vi "LifeTesting.vi"() -> ()   [LabVIEW 2016]
uses:
  <vilib>/Instr/_visa.llb/VISA Configure Serial Port (Instr).vi
  <vilib>/Utility/config.llb/Read Key (Double).vi
  <vilib>/Utility/file.llb/Write Delimited Spreadsheet (DBL).vi
  <vilib>/Utility/config.llb/NI_LVConfig.lvlib
panel:
  in  "两次测量间工作次数":i32=44
  in  "osc chn":i32[](array[numeric])
  in  "总共需要测量次数":i32
  out "轴向声压分布":cluster{dbl[], dbl[]}(graph)
  in  "sensitivity":dbl=0.2
  out "preasure":dbl
  in  "record cycles":dbl=7.0
  in  "freq (MHz)":dbl=1.367
  in  "cycles":dbl=60.0
  in  "Port":u32=12321
  in  "HIFU IP":string="192.168.1.24"
  in  "探头测量中心位置":dbl[][](array[numeric])
  in  "KYCT":refnum<visa-resource-name>
  in  "osc in":refnum<visa-resource-name>
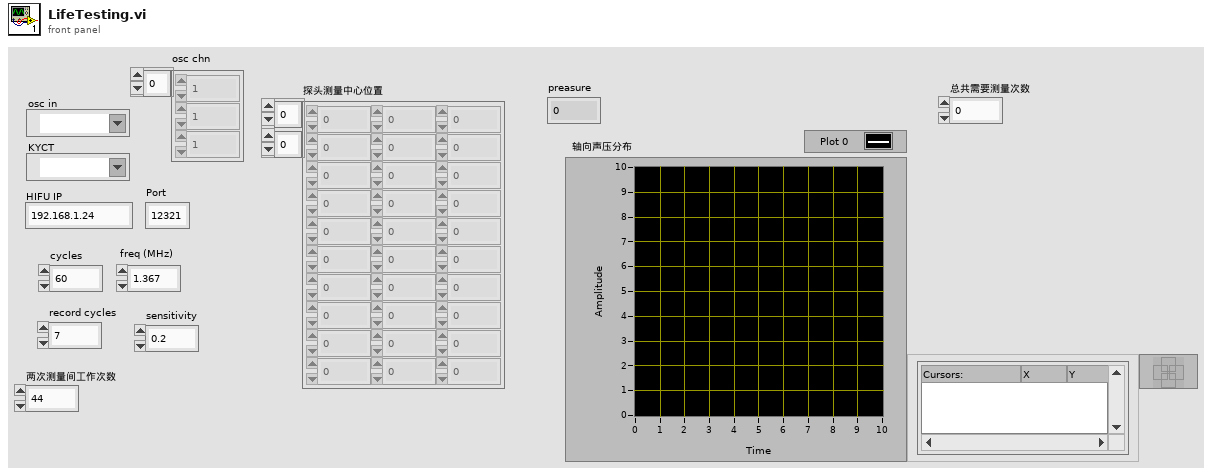
[diagram p1: front panel]
types:
  T1 = typedef "NI_LVConfig.lvlib/Config Data RefNum.ctl" = refnum<k1>
  T2 = typedef "NI_Matrix.lvlib/RealMatrix.ctl" = dbl[][]
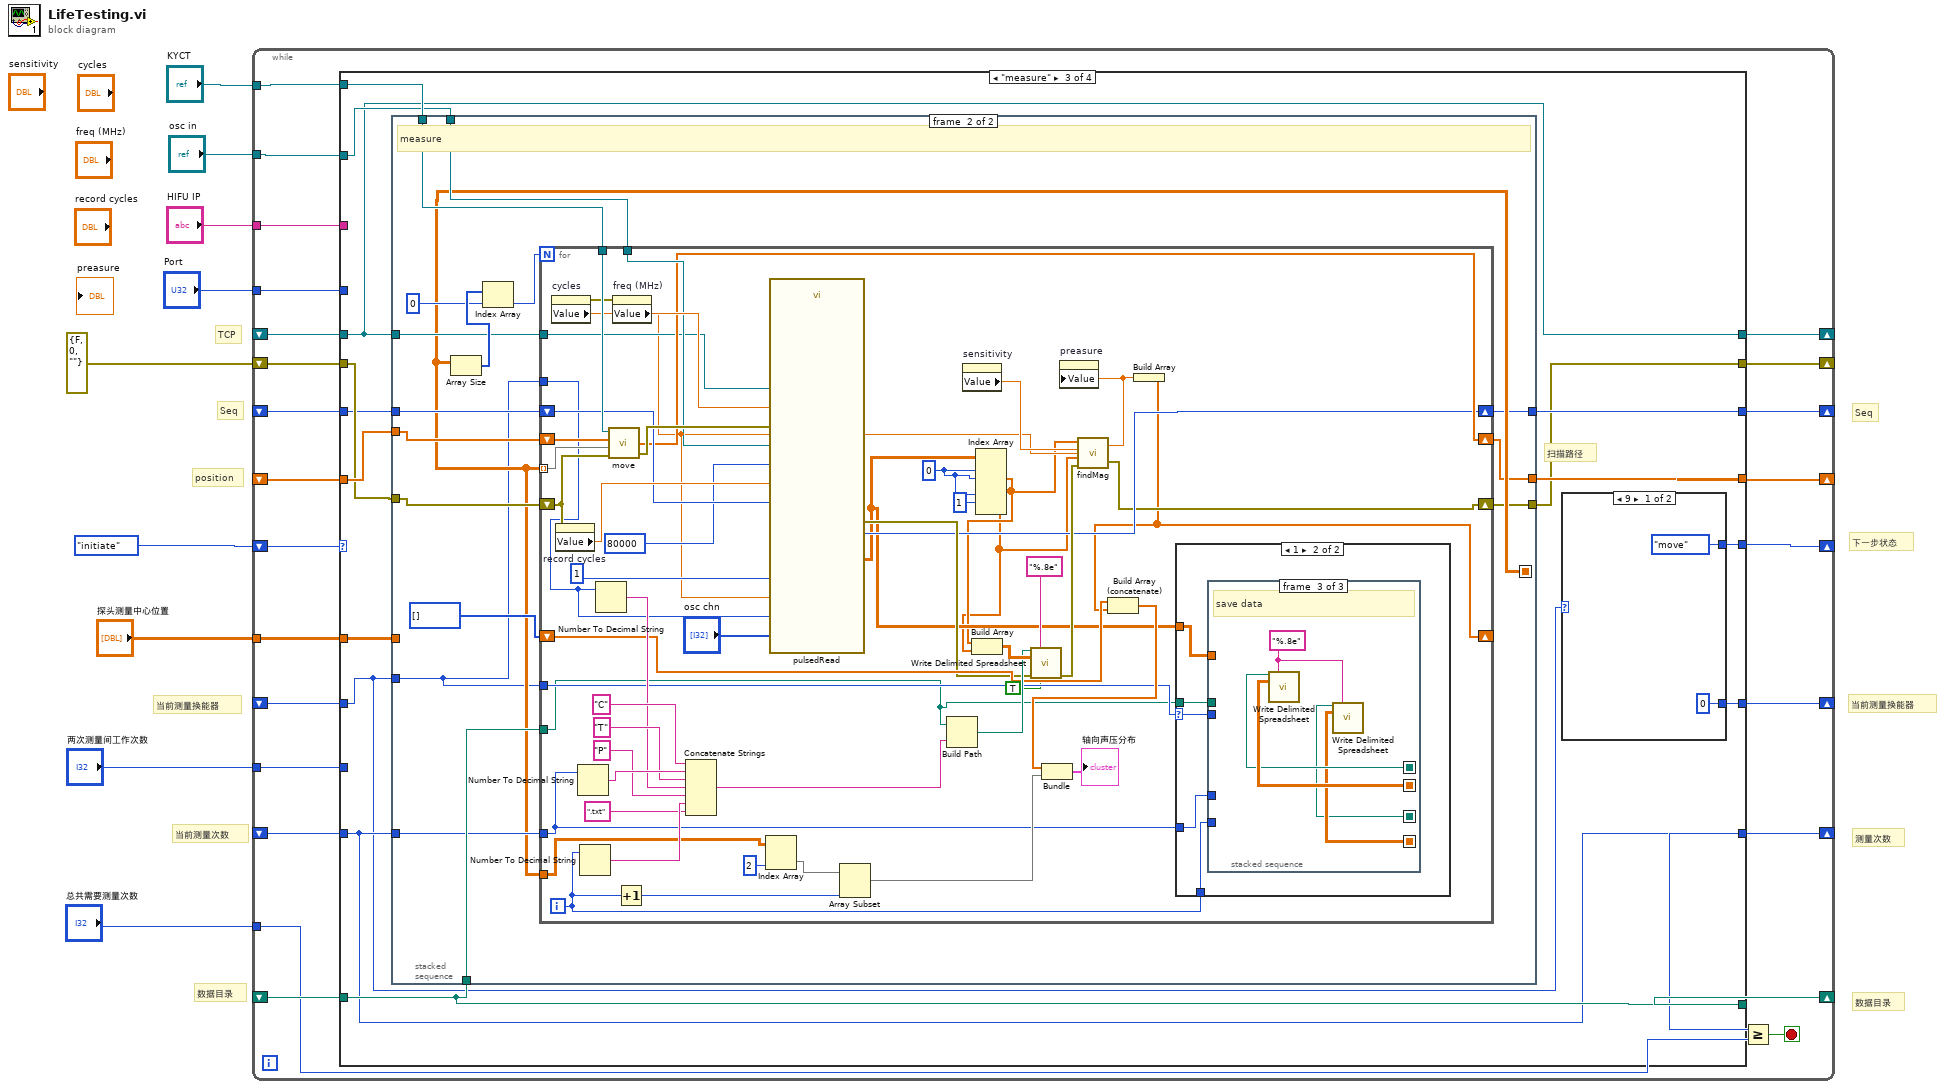
[diagram p0: block diagram]
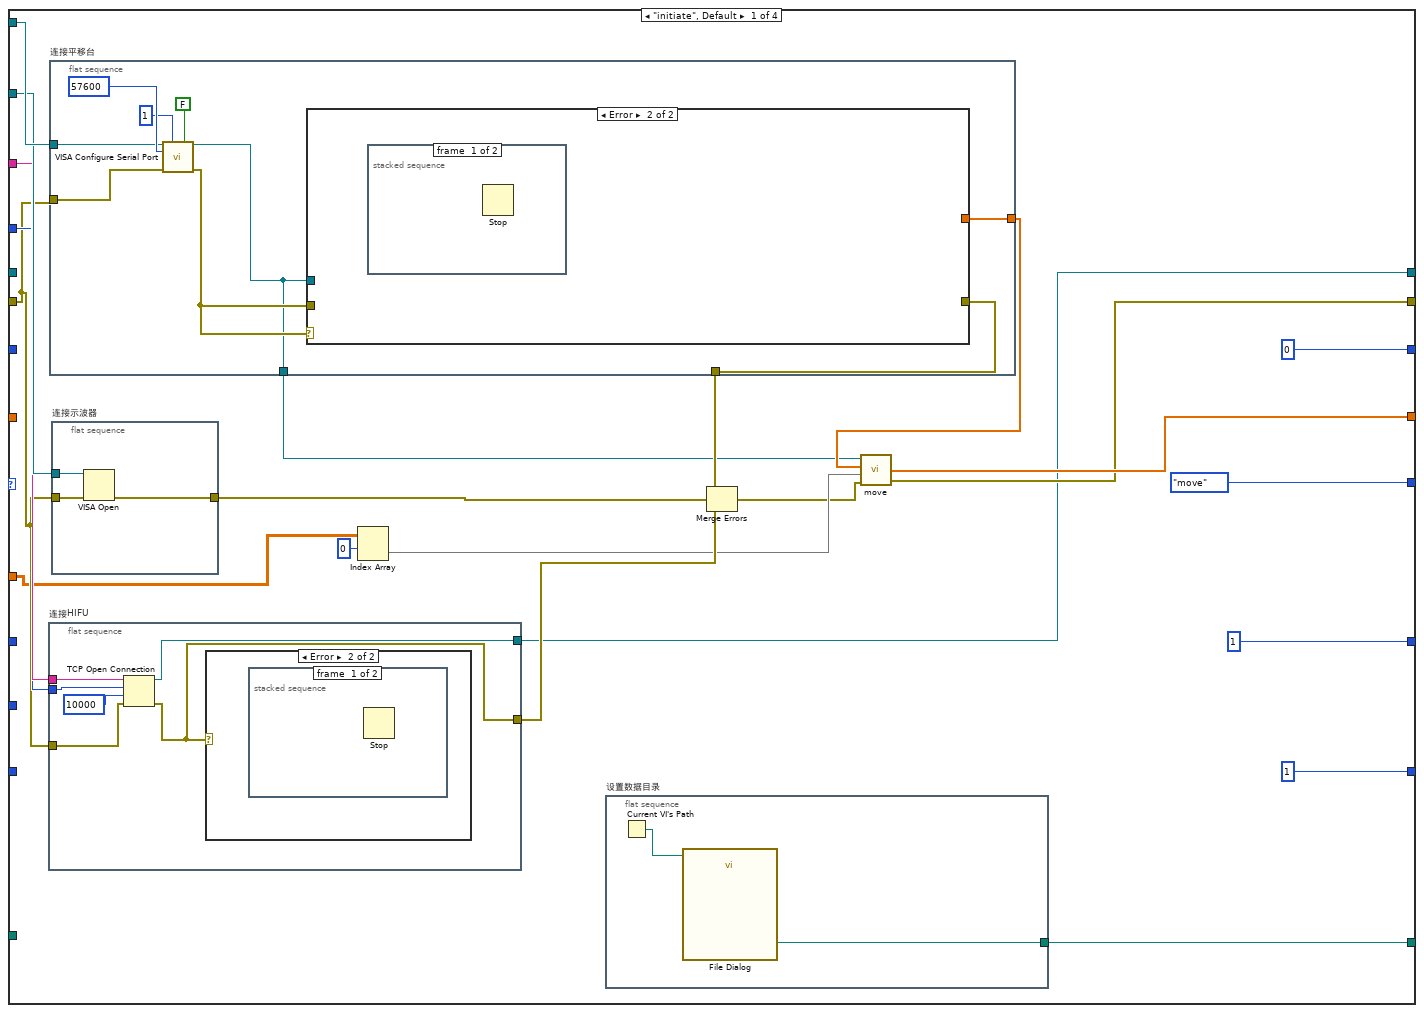
[diagram p2: hidden frame]
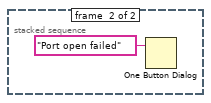
[diagram p4: hidden frame]
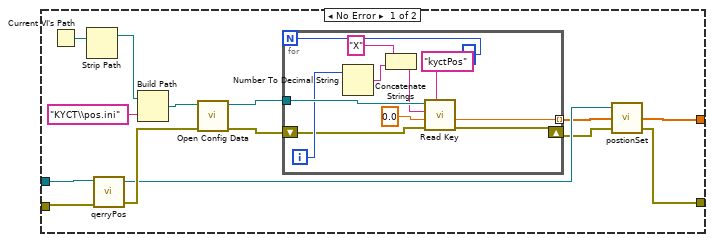
[diagram p5: hidden frame]
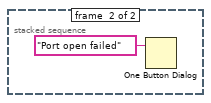
[diagram p6: hidden frame]
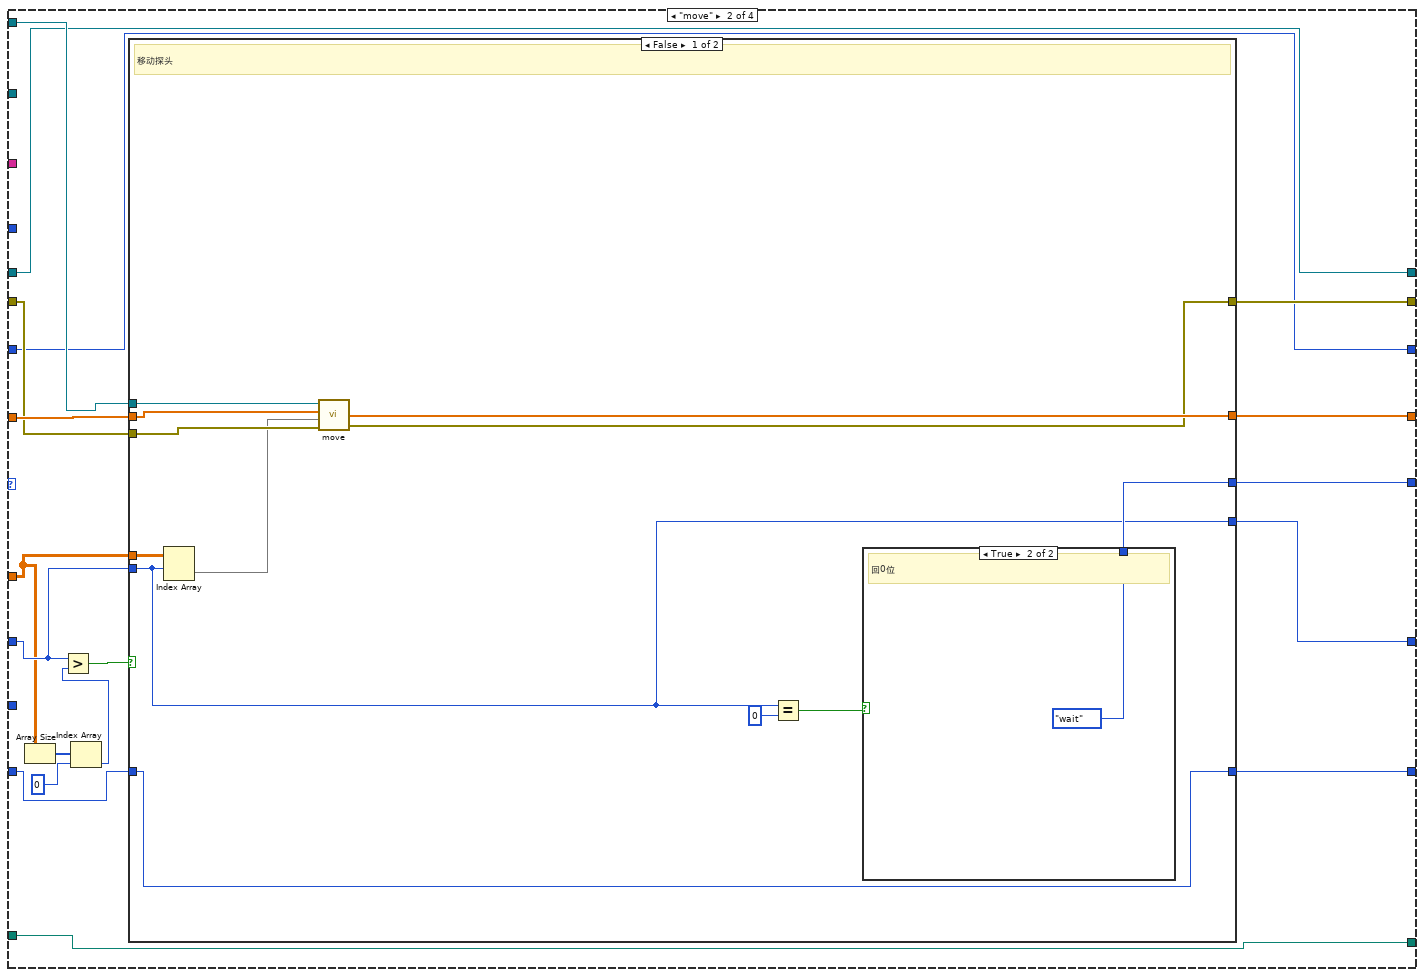
[diagram p7: hidden frame]
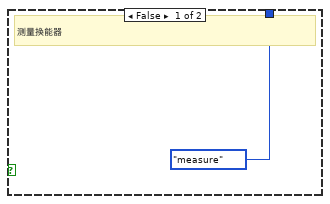
[diagram p8: hidden frame]
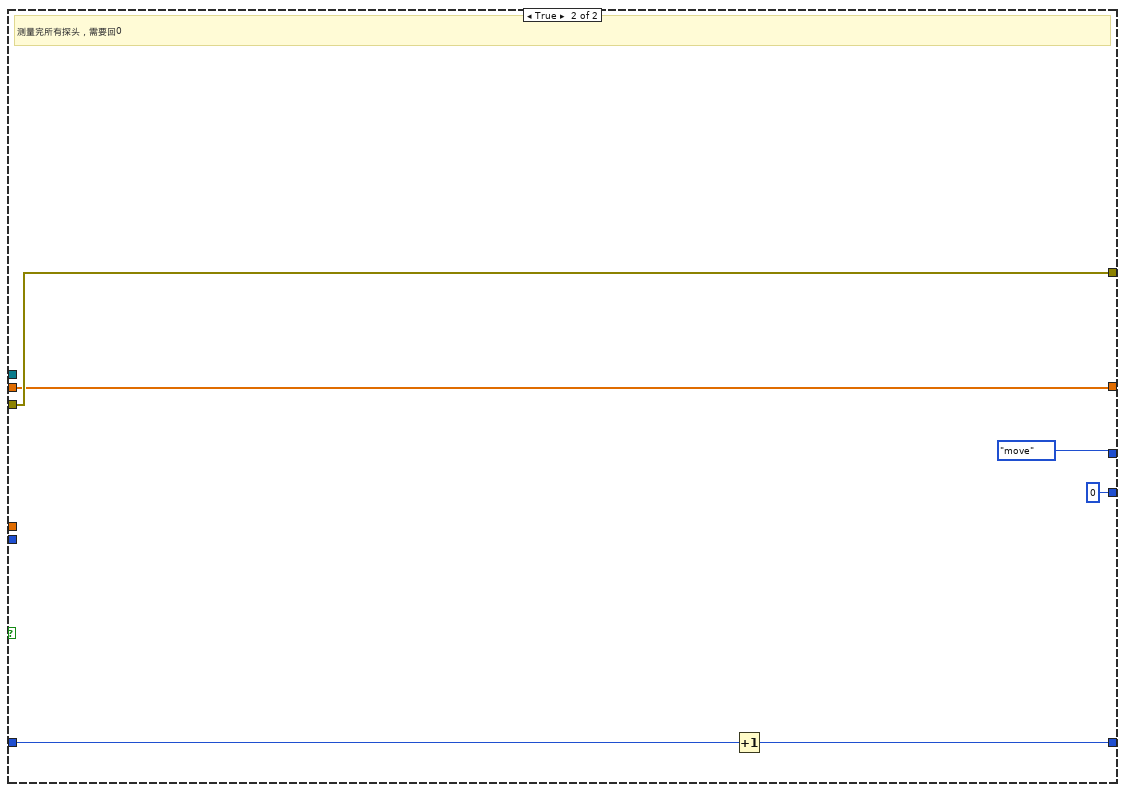
[diagram p9: hidden frame]
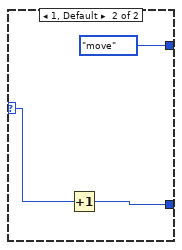
[diagram p10: hidden frame]
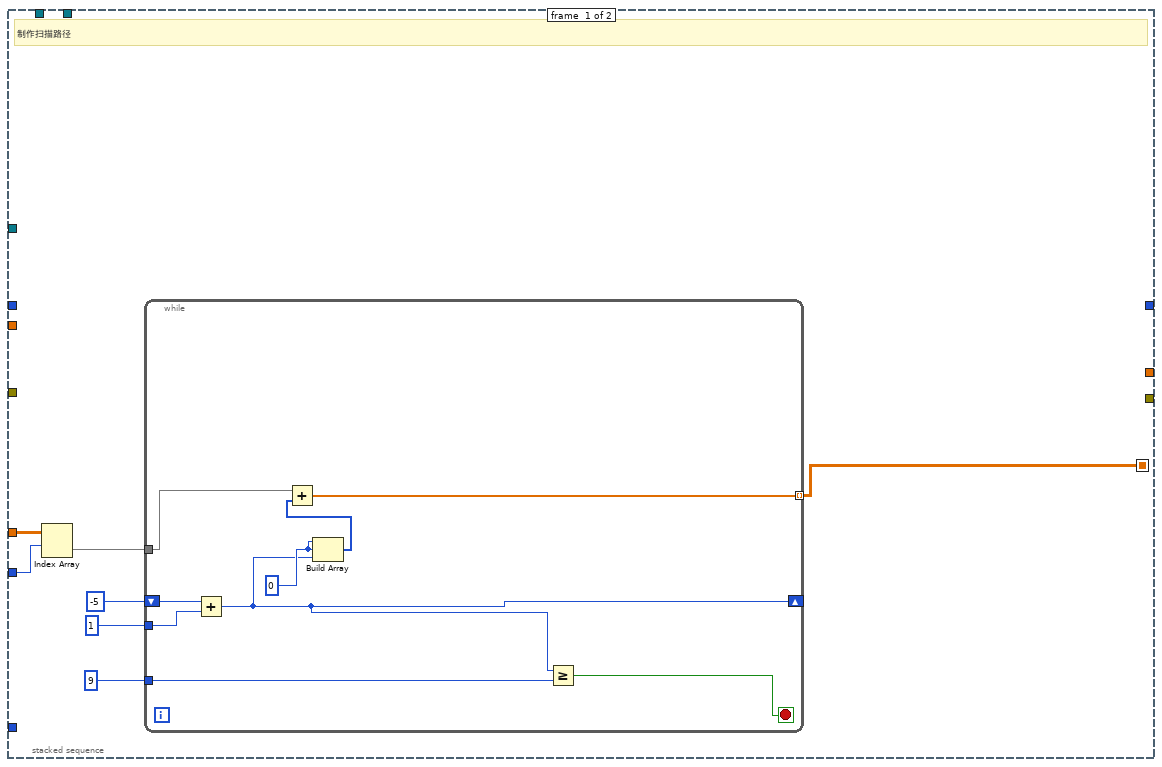
[diagram p11: hidden frame]
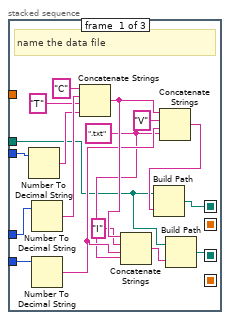
[diagram p13: hidden frame]
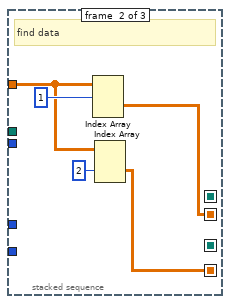
[diagram p14: hidden frame]
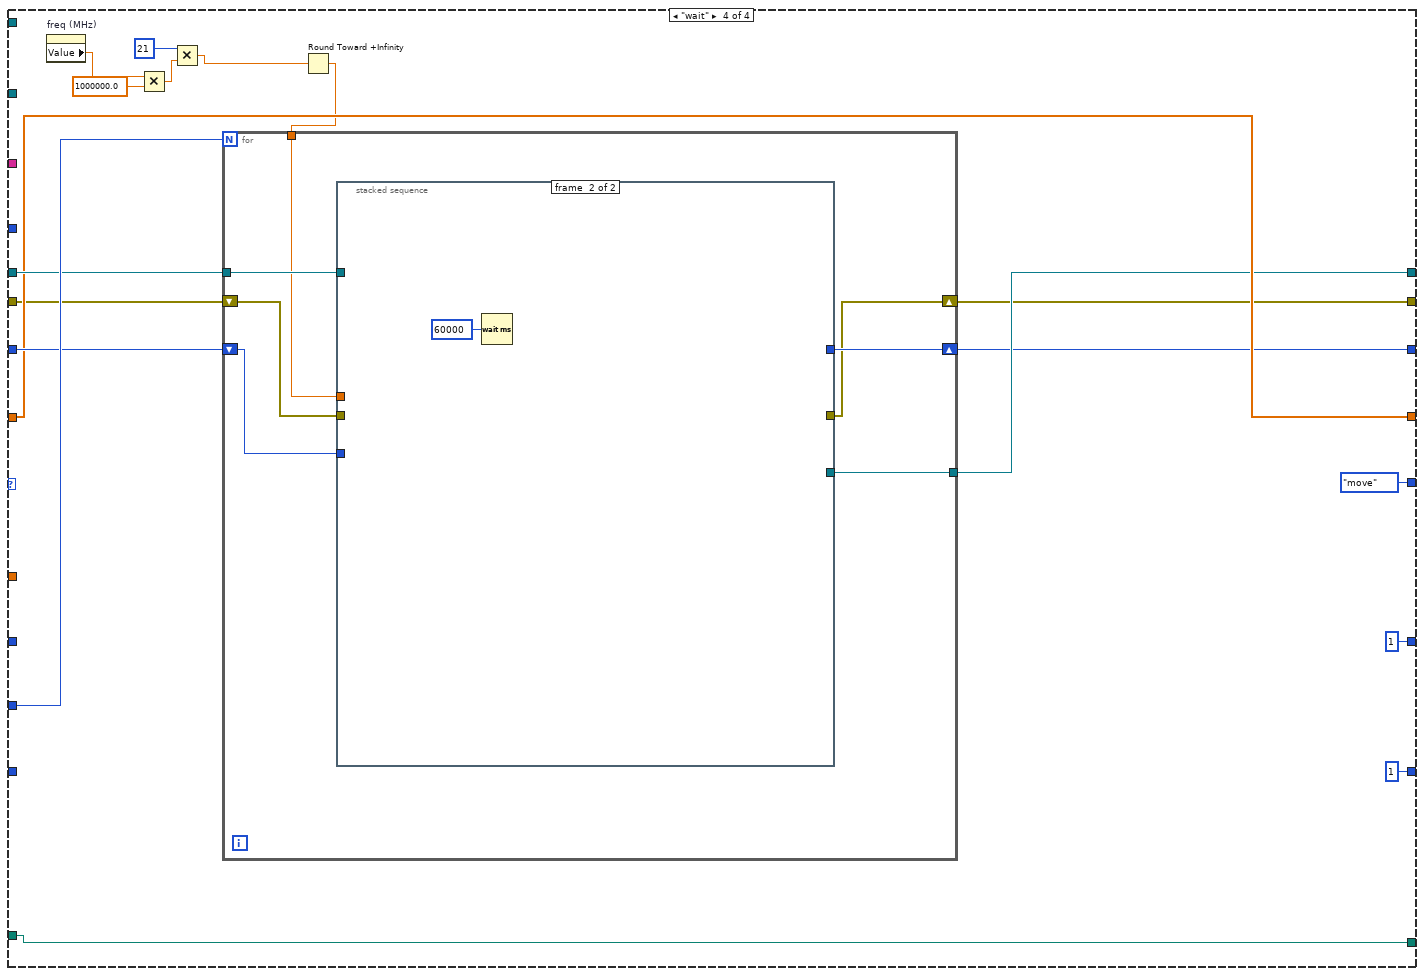
[diagram p15: hidden frame]
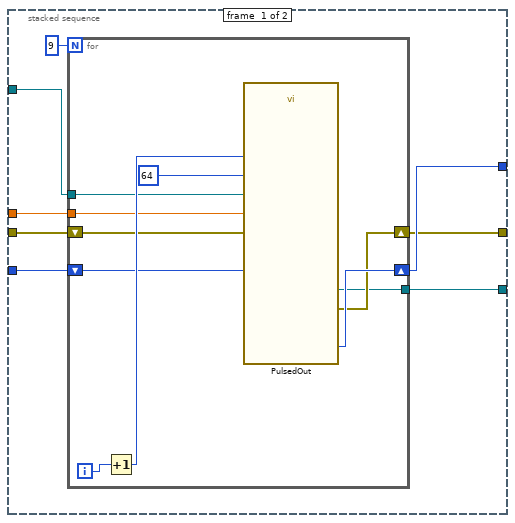
[diagram p16: hidden frame]
diagram:
  # "Seq"
  # "当前测量次数"
  # "数据目录"
  # "测量次数"
  # "Seq"
  # "数据目录"
  # "当前测量换能器"
  # "下一步状态"
  # "当前测量换能器"
  # "TCP"
  # "position"
  n1 = while {
    shift-right: [w32] -> _
    shift-left: errorcluster {"status"=FALSE, "code"=0, "source"=""} ("error constant") -> [w29]
    tunnel: "KYCT" -> [w31]
    tunnel: "osc in" -> [w30]
    tunnel: "HIFU IP" -> [w28]
    tunnel: "Port" -> [w27]
    shift-right: [w26] -> _
    shift-left: enum16{"initiate", "move", "measure", "wait"}."initiate" -> [w33]
    shift-right: [w25] -> _
    shift-left: _ -> [w24]
    shift-right: [w17] -> _
    shift-left: _ -> [w16]
    tunnel: "探头测量中心位置" -> [w23]
    shift-right: [w20] -> _
    shift-left: _ -> [w22]
    shift-right: [w13] -> _
    shift-left: _ -> [w21]
    shift-right: [w18] -> _
    shift-left: _ -> [w19]
    shift-right: [w15] -> _
    shift-left: _ -> [w14]
    tunnel: "总共需要测量次数" -> [w12]
    tunnel: "两次测量间工作次数" -> [w10]
    stop <- w11 stop-if-true
    n2 = case shown="\"measure\"" w33 {
      tunnel: w29 -> [w48 w117 w152 w285]
      tunnel: [w39 w114 w147 w283] -> w32
      tunnel: w31 -> [w55 w119 w153 _]
      tunnel: w30 -> [w54 _ w151 _]
      tunnel: w28 -> [w53 _ _ _]
      tunnel: w27 -> [w52 _ _ _]
      tunnel: [enum16{"initiate", "move", "measure", "wait"}."move" w113 w146 enum16{"initiate", "move", "measure", "wait"}."move"] -> w26
      tunnel: [w40 w115 w149 w292] -> w25
      tunnel: w24 -> [_ w118 w154 w292]
      tunnel: w23 -> [w44 w111 w155 _]
      tunnel: w22 -> [_ w116 w141 _]
      tunnel: w21 -> [_ w107 w143 _]
      tunnel: [1 w112 w145 1] -> w20
      tunnel: [1 w106 w143 1] -> w13
      tunnel: w19 -> [_ w105 w150 w293]
      tunnel: [u32 0 ("SEQ OUT") w105 w148 w282] -> w18
      tunnel: [w37 w104 w142 w284] -> w17
      tunnel: w16 -> [_ w104 w142 w294]
      tunnel: [w36 w103 w144 w296] -> w15
      tunnel: w14 -> [_ w103 w144 w296]
      tunnel: w10 -> [_ _ _ w295]
      frame "initiate", Default {
        n3 = flat-sequence "连接HIFU" {
          tunnel: w53 -> [w63]
          tunnel: w52 -> [w62]
          tunnel: w48 -> [w60]
          tunnel: [w59] -> w49
          tunnel: [w58] -> w37
          frame #0 {
            n4 = TCP Open Connection(address=w63, remote port or service name=w62, timeout ms (60000)=10000, error in (no error)=w60) -> (connection ID=w58:refnum<k5>, error out=w59:errorcluster)  [unwired: 1 in]
            n5 = case shown="Error" w59 {
              frame No Error {
              }
              frame Error {
                n6 = stacked-sequence {
                  frame #0 {
                    n7 = Stop() -> ()  [unwired: 1 in]
                  }
                  frame #1 {
                    n8 = One Button Dialog(message="Port open failed") -> ()  [unwired: 1 in, 1 out]
                  }
                }
              }
            }
          }
        }
        n9 = flat-sequence "连接平移台" {
          tunnel: w48 -> [w73]
          tunnel: [w71] -> w51
          tunnel: w55 -> [w70]
          tunnel: [w69] -> w46
          tunnel: [w68] -> w45
          frame #0 {
            n10 = call-poly "VISA Configure Serial Port"("VISA resource name"=w70, "timeout (10sec)"=u32 1, "Enable Termination\nChar (T)"=FALSE ("Enable Termination\nChar (T)"), "baud rate (9600)"=u32 57600, "error in (no error)"=w73) -> ("VISA resource name out"=w68:refnum<visa-resource-name>, "error out"=w72:errorcluster)  [unwired: 9 in]
            n11 = case shown="Error" w72 {
              tunnel: w68 -> [w91 _]
              tunnel: [w79 _] -> w69
              tunnel: w72 -> [w78 _]
              tunnel: [w77 _] -> w71
              frame No Error {
                n12 = Current VI's Path() -> (path=w90:path)
                n13 = Strip Path(path=w90) -> (stripped path=w89:path)  [unwired: 1 out]
                n14 = call "qerryPos.vi"("error in (no error)"=w78, "UART in"=w91) -> ("error out"=w86:errorcluster, "UART out"=w82:refnum<visa-resource-name>)  [unwired: 2 in, 1 out]
                n15 = Build Path(base path=w89, name or relative path="KYCT\\pos.ini") -> (appended path=w87:path)
                n16 = call <vilib>:"Open Config Data.vi"("error in (no error)"=w86, "configuration file path"=w87) -> ("error out"=w84:errorcluster, "refnum"=w83:T1)  [unwired: 7 in, 1 out]
                n17 = for {
                  N: 3 -> [_]
                  tunnel: w83 -> [w101]
                  shift-right: [w94] -> w81
                  shift-left: w84 -> [w95]
                  tunnel: [w93] -> w80 mode=indexing
                  i -> [w97]
                  n18 = Number To Decimal String(number=w97) -> (decimal integer string=w99:string)  [unwired: 1 in]
                  n19 = Concatenate Strings("X" ("string"), w99) -> (w98:string)
                  n20 = call-poly <vilib>:"Read Key.vi"("section"="kyctPos", "error in (no error)"=w95, "default value"=0.0, "key"=w98, "refnum"=w101) -> ("error out"=w94:errorcluster, "value"=w93:dbl)  [unwired: 3 in, 2 out]
                }
                n21 = call "postionSet.vi"("error in (no error)"=w81, "Pos in"=w80, "UART PORT in"=w82) -> ("error out"=w77:errorcluster, "Pos out"=w79:dbl[])  [unwired: 1 out]
              }
              frame Error {
                n22 = stacked-sequence {
                  frame #0 {
                    n23 = Stop() -> ()  [unwired: 1 in]
                  }
                  frame #1 {
                    n24 = One Button Dialog(message="Port open failed") -> ()  [unwired: 1 in, 1 out]
                  }
                }
              }
            }
          }
        }
        n25 = flat-sequence "连接示波器" {
          tunnel: w54 -> [w67]
          tunnel: w48 -> [w66]
          tunnel: [w65] -> w50
          frame #0 {
            n26 = VISA Open(error in (no error)=w66, VISA resource name=w67) -> (error out=w65:errorcluster)  [unwired: 3 in, 1 out]
          }
        }
        n27 = Index Array(array=w44, index (row)=0) -> (element=w42:dbl[])  [unwired: 1 in]
        n28 = flat-sequence "设置数据目录" {
          tunnel: [w56] -> w36
          frame #0 {
            n29 = Current VI's Path() -> (path=w57:path)
            n30 = call "File Dialog"("start path"=w57) -> ("selected path"=w56:path)  [unwired: 11 in, 3 out]
          }
        }
        n31 = Merge Errors(w51, w50, w49) -> (w41:errorcluster)
        n32 = call "move.vi"("error in (no error)"=w41, "P01"=w42, "P0"=w46, "UART PORT in"=w45) -> ("error out"=w39:errorcluster, "P1"=w40:dbl[])  [unwired: 1 out]
      }
      frame "move" {
        n33 = Array Size(array=w111) -> (size(s)=w110:i32[])
        n34 = Index Array(array=w110, index=0) -> (element=w108:i32)
        n35 = Greater?(x=w116, y=w108) -> (0:w120:bool)
        n36 = case shown="False" w120 {
          tunnel: w119 -> [w132 _]
          tunnel: w118 -> [w131 w137]
          tunnel: w117 -> [w130 w140]
          tunnel: w116 -> [w122 _]
          tunnel: w111 -> [w129 _]
          tunnel: [w127 w137] -> w115
          tunnel: [w126 w140] -> w114
          tunnel: [w123 enum16{"initiate", "move", "measure", "wait"}."move"] -> w113
          tunnel: [w122 0] -> w112
          tunnel: w107 -> [w121 w136]
          tunnel: [w121 w135] -> w106
          frame False {
            # "移动探头"
            n37 = Index Array(array=w129, index (row)=w122) -> (element=w128:dbl[])  [unwired: 1 in]
            n38 = call "move.vi"("error in (no error)"=w130, "P01"=w128, "P0"=w131, "UART PORT in"=w132) -> ("error out"=w126:errorcluster, "P1"=w127:dbl[])  [unwired: 1 out]
            n39 = Equal?(x=w122, y=0) -> (x = y?=w124:bool)
            n40 = case shown="True" w124 {
              tunnel: [enum16{"initiate", "move", "measure", "wait"}."measure" enum16{"initiate", "move", "measure", "wait"}."wait"] -> w123
              frame False {
                # "测量换能器"
              }
              frame True {
                # "回0位"
              }
            }
          }
          frame True {
            # "测量完所有探头，需要回0"
            n41 = Increment(x=w136) -> (x+1=w135:i32)
          }
        }
      }
      frame "measure" {
        # "扫描路径"
        n42 = stacked-sequence {
          seq-local: [w162 _] -> [_ w181]
          tunnel: w155 -> [w167 _]
          tunnel: w141 -> [w166 w177]
          tunnel: w154 -> [_ w190]
          tunnel: w153 -> [_ w189]
          tunnel: w152 -> [_ w188]
          tunnel: w151 -> [_ w187]
          tunnel: w150 -> [_ w186]
          tunnel: w142 -> [_ w185]
          tunnel: w144 -> [_ w184]
          tunnel: w143 -> [_ w183]
          tunnel: [_ w180] -> w149
          tunnel: [_ w179] -> w148
          tunnel: [_ w178] -> w147
          frame #0 {
            # "制作扫描路径"
            n43 = Index Array(array=w167, index (row)=w166) -> (element=w165:dbl[])  [unwired: 1 in]
            n44 = while {
              tunnel: w165 -> [w173]
              tunnel: 1 -> [w175]
              shift-right: [w170] -> _
              shift-left: -5 -> [w176]
              tunnel: [w171] -> w162 mode=indexing
              tunnel: 9 ("y") -> [w168]
              stop <- w169 stop-if-true
              w174 = 0 ("element")
              n45 = Add(x=w176, y=w175) -> (x+y=w170:i32)
              n46 = Build Array(w174, w174, w170) -> (w172:i32[])
              n47 = Add(x=w173, y=w172) -> (x+y=w171:dbl[])
              n48 = Greater Or Equal?(x=w170, y=w168) -> (x >= y?=w169:bool)
            }
          }
          frame #1 {
            # "measure"
            n49 = Array Size(array=w181) -> (size(s)=w193:i32[])
            n50 = Index Array(array=w193, index=0) -> (element=w192:i32)
            n51 = for {
              N: w192 -> [_]
              tunnel: w181 -> [w245] mode=indexing
              tunnel: w189 -> [w244]
              tunnel: w177 -> [w213]
              tunnel: w187 -> [w240]
              tunnel: w185 -> [w212]
              tunnel: w184 -> [w197]
              tunnel: w183 -> [w198]
              shift-right: [w202] -> _
              shift-left: i32[] [] -> [w223]
              tunnel: w181 -> [w221]
              shift-right: [w203] -> w178
              shift-left: w188 -> [w239]
              shift-right: [w215] -> w180
              shift-left: w190 -> [w246]
              shift-right: [w204] -> w179
              shift-left: w186 -> [w237]
              tunnel: w177 -> [w201]
              i -> [w199]
              w208 = 0 ("index (page)")
              n52 = property on="cycles" class="DigNum (strict)"() -> (error out=w241:errorcluster, "Value"=w243:dbl)  [unwired: 2 in, 1 out]
              n53 = property on="record cycles" class="DigNum (strict)"(error in=w239) -> ("Value"=w238:dbl)  [unwired: 1 in, 2 out]
              n54 = Number To Decimal String(number=w198) -> (decimal integer string=w235:string)  [unwired: 1 in]
              n55 = Number To Decimal String(number=w199) -> (decimal integer string=w231:string)  [unwired: 1 in]
              n56 = Number To Decimal String(number=w213) -> (decimal integer string=w233:string)  [unwired: 1 in]
              n57 = call "move.vi"("error in (no error)"=w239, "P01"=w245, "P0"=w246, "UART PORT in"=w244) -> ("error out"=w242:errorcluster, "P1"=w215:dbl[])  [unwired: 1 out]
              n58 = property on="freq (MHz)" class="DigNum (strict)"(error in=w241) -> ("Value"=w210:dbl)  [unwired: 1 in, 2 out]
              n59 = Increment(x=w199) -> (x+1=w218:i32)
              n60 = Concatenate Strings("C", w235, "T" ("element"), w233, "P" ("element"), w231, ".txt" ("element")) -> (w229:string)
              n61 = Index Array(array=w221, index (col)=2 ("disabled index (col)")) -> (element=w219:dbl[])  [unwired: 1 in]
              n62 = call "pulsedRead.vi"("connection ID"=w212, "osc in"=w240, "freq"=w210, "recCycles"=w238, "SEQ IN"=w237, "cycles"=w243, "error in (no error)"=w242, "osc chn"="osc chn", "points"=u64 80000, "chn num"=1 ("osc channel"), "HIFU chn"=w213) -> ("time&voltage"=w200:dbl[][][], "error out"=w209:errorcluster, "SEQ OUT"=w204:u32)  [unwired: 2 in]
              n63 = Array Subset(array=w219, length=w218) -> (w217:dbl[])  [unwired: 1 in]
              n64 = Build Path(base path=w197, name or relative path=w229) -> (appended path=w227:path)
              n65 = property on="sensitivity" class="DigNum (strict)"() -> ("Value"=w224:dbl)  [unwired: 2 in, 2 out]
              n66 = Index Array(array=w200, index (dim 0) #1=w208, index (dim 1) #1=w208, index (dim 0) #2=w208, index (dim 1) #2=1 ("disabled index (row)")) -> (element #1=w195:dbl[], element #2=w194:dbl[])  [unwired: 2 in]
              n67 = Build Array(w195, w194) -> (w228:T2)
              n68 = call-poly <vilib>:"Write Delimited Spreadsheet.vi"("file path (dialog if empty)"=w227, "format (%.3f)"="%.8e", "2D data"=w228, "error in (no error)"=w209, "transpose? (no:F)"=TRUE) -> ("error out"=w225:errorcluster)  [unwired: 9 in, 1 out]
              n69 = call "findMag.vi"("times"=w195, "sens"=w224, "voltages"=w194, "error in (no error)"=w225, "freq"=w210) -> ("magfound"=w222:dbl, "error out"=w203:errorcluster)
              n70 = property on="preasure" class="DigNum (strict)"("Value"=w222) -> ()  [unwired: 2 in, 2 out]
              n71 = Build Array(w222) -> (w202:dbl[])
              n72 = Build Array (concatenate)(w223, w202) -> (w205:dbl[])
              n73 = Bundle(w205, w217) -> (→"轴向声压分布":cluster{dbl[], dbl[]})  [unwired: 1 in]
              n74 = case shown="1" w201 {
                selector: w201 -> [_ w249]
                tunnel: w200 -> [_ w247]
                tunnel: w199 -> [_ w251]
                tunnel: w198 -> [_ w250]
                tunnel: w197 -> [_ w248]
                frame 0, Default {
                }
                frame 1 {
                  n75 = stacked-sequence {
                    seq-local: [w259 _ _] -> [_ _ w277]
                    seq-local: [w252 _ _] -> [_ _ w274]
                    seq-local: [_ w270 _] -> [_ _ w278]
                    seq-local: [_ w269 _] -> [_ _ w275]
                    tunnel: w251 -> [w262 _ _]
                    tunnel: w250 -> [w267 _ _]
                    tunnel: w249 -> [w264 _ _]
                    tunnel: w248 -> [w254 _ _]
                    tunnel: w247 -> [_ w272 _]
                    frame #0 {
                      w255 = ".txt" ("string")
                      # "name the data file"
                      n76 = Number To Decimal String(number=w264) -> (decimal integer string=w263:string)  [unwired: 1 in]
                      n77 = Number To Decimal String(number=w267) -> (decimal integer string=w266:string)  [unwired: 1 in]
                      n78 = Number To Decimal String(number=w262) -> (decimal integer string=w256:string)  [unwired: 1 in]
                      n79 = Concatenate Strings("C" ("string"), w266, "T" ("string"), w263) -> (w258:string)
                      n80 = Concatenate Strings(w258, "I" ("string"), w256, w255) -> (w253:string)
                      n81 = Concatenate Strings(w258, "V" ("string"), w256, w255) -> (w260:string)
                      n82 = Build Path(base path=w254, name or relative path=w260) -> (appended path=w259:path)
                      n83 = Build Path(base path=w254, name or relative path=w253) -> (appended path=w252:path)
                    }
                    frame #1 {
                      # "find data"
                      n84 = Index Array(array=w272, index (dim 0)=1 ("index (page)")) -> (element=w270:dbl[][])  [unwired: 2 in]
                      n85 = Index Array(array=w272, index (dim 1)=2 ("disabled index (row)")) -> (element=w269:dbl[][])  [unwired: 2 in]
                    }
                    frame #2 {
                      w276 = "%.8e" ("format (%.3f)")
                      # "save data"
                      n86 = call-poly <vilib>:"Write Delimited Spreadsheet.vi"("file path (dialog if empty)"=w277, "format (%.3f)"=w276, "2D data"=w278) -> ()  [unwired: 11 in, 2 out]
                      n87 = call-poly <vilib>:"Write Delimited Spreadsheet.vi"("file path (dialog if empty)"=w274, "format (%.3f)"=w276, "2D data"=w275) -> ()  [unwired: 11 in, 2 out]
                    }
                  }
                }
              }
            }
          }
        }
        n88 = case shown="9" w141 {
          selector: w141 -> [_ w158]
          tunnel: [enum16{"initiate", "move", "measure", "wait"}."move" enum16{"initiate", "move", "measure", "wait"}."move"] -> w146
          tunnel: [0 w159] -> w145
          frame 9 {
          }
          frame 1, Default {
            n89 = Increment(x=w158) -> (x+1=w159:i32)
          }
        }
      }
      frame "wait" {
        n90 = property on="freq (MHz)" class="DigNum (strict)"() -> ("Value"=w290:dbl)  [unwired: 2 in, 2 out]
        n91 = Multiply(x=w290, y=1000000.0) -> (x*y=w288:dbl)
        n92 = Multiply(x=21, y=w288) -> (x*y=w287:dbl)
        n93 = Round Toward +Infinity(x=w287) -> (ceil(x): smallest int >= x=w286:dbl)
        n94 = for {
          N: w295 -> [_]
          tunnel: w294 -> [w303]
          shift-right: [w299] -> w282
          shift-left: w293 -> [w301]
          tunnel: w286 -> [w302]
          shift-right: [w298] -> w283
          shift-left: w285 -> [w300]
          tunnel: [w297] -> w284
          n95 = stacked-sequence {
            tunnel: w303 -> [w310 _]
            tunnel: w302 -> [w309 _]
            tunnel: w301 -> [w308 _]
            tunnel: w300 -> [w307 _]
            tunnel: [w306 _] -> w299
            tunnel: [w305 _] -> w298
            tunnel: [w304 _] -> w297
            frame #0 {
              n96 = for {
                N: 9 -> [_]
                tunnel: w310 -> [w318]
                tunnel: w309 -> [w317]
                shift-right: [w315] -> w306
                shift-left: w308 -> [w316]
                shift-right: [w313] -> w305
                shift-left: w307 -> [w314]
                tunnel: [w312] -> w304
                i -> [w321]
                n97 = Increment(x=w321) -> (x+1=w320:i32)
                n98 = call "PulsedOut.vi"("Cycles"=w317, "Channel"=w320, "error in (no error)"=w314, "SEQ IN"=w316, "chn num"=u16 64, "connection ID"=w318) -> ("error out"=w313:errorcluster, "connection ID out"=w312:refnum<k5>, "SEQ OUT"=w315:u32)  [unwired: 1 in, 1 out]
              }
            }
            frame #1 {
              n99 = Wait (ms)(milliseconds to wait=u32 60000) -> ()  [unwired: 1 out]
            }
          }
        }
      }
    }
    n100 = Greater Or Equal?(x=w13, y=w12) -> (x >= y?=w11:bool)
  }
